vi "failUnlessXmlParsedCorrectly.vi"(4 "Convert EOL? (TRUE)":bool=TRUE, 6 "message (\"\")":string, 8 "error in":errorcluster, 9 "Expected Data":variant, 10 "XML String":string, 11 "reference in":refnum<class "EasyXML_XML_Subset_Evaluations.lvclass">) -> (0 "error out":errorcluster, 2 "Produced Data":variant, 3 "reference in":refnum<class "EasyXML_XML_Subset_Evaluations.lvclass">)   [LabVIEW 2013, in "EasyXML_XML_Subset_Evaluations.lvclass"]
doc: "Tests whether an XML string input matches flattened XML output generated from an in data structure"
uses:
  EasyXML_XML_Subset_Evaluations.lvclass
panel:
  # "Copyright © 2007 James Kring, Inc. All rights reserved.\n\nAuthor: Jim Kring [jim.kring@jameskring.com]\n\nThis library is provided \"AS IS\" ,WITHOUT WARRANTIES OR \nCONDITIONS OF ANY KIND, either express or implied.\n\nJames Kring, Inc. -- http://www.jameskring.com"
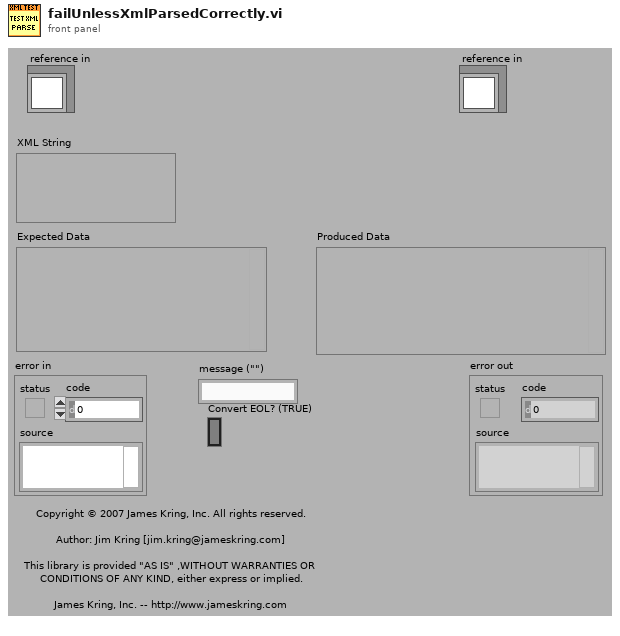
[diagram p1: front panel]
types:
  T1 = typedef "Type Descriptor__ogtk.ctl" = i16[]
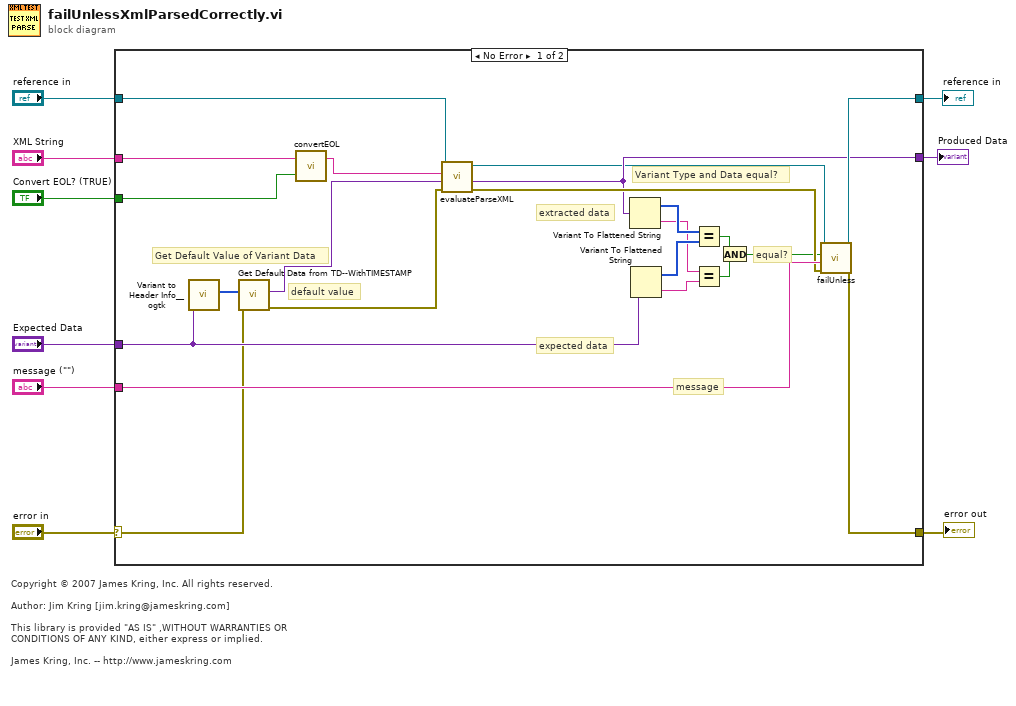
[diagram p0: block diagram]
diagram:
  # "Copyright © 2007 James Kring, Inc. All rights reserved.\n\nAuthor: Jim Kring [jim.kring@jameskring.com]\n\nThis library is provided \"AS IS\" ,WITHOUT WARRANTIES OR \nCONDITIONS OF ANY KIND, either express or implied.\n\nJames Kring, Inc. -- http://www.jameskring.com"
  n1 = case shown="No Error" "error in" {
    selector: "error in" -> [w12 w33]
    tunnel: [w26 w33] -> w8
    tunnel: [w28 w32] -> w6
    tunnel: "reference in" -> [w11 w32]
    tunnel: "message (\"\")" -> [w31 _]
    tunnel: "Expected Data" -> [w14 _]
    tunnel: "XML String" -> [w25 _]
    tunnel: [w22 _] -> w2
    tunnel: "Convert EOL? (TRUE)" -> [w23 _]
    frame No Error {
      # "Variant Type and Data equal?"
      # "message"
      # "equal?"
      # "expected data"
      # "extracted data"
      # "Get Default Value of Variant Data"
      # "default value"
      n2 = call <userlib>:"Variant to Header Info__ogtk.vi"("Variant"=w14) -> ("Type Descriptor"=w13:T1)  [unwired: 3 in, 2 out]
      n3 = call "Get Default Data from TD--WithTIMESTAMP.vi"("error in"=w12, "Type Descriptor"=w13) -> ("error out"=w30:errorcluster, "Default VData"=w29:variant)  [unwired: 8 in]
      n4 = call "convertEOL.vi"("Convert EOL? (TRUE)"=w23, "string"=w25) -> ("string out"=w24:string)  [unwired: 1 in]
      n5 = call-dynamic "evaluateParseXML.vi"("error in"=w30, "Default VData"=w29, "XML string"=w24, "reference in"=w11) -> ("error out"=w27:errorcluster, "LabVIEW Data"=w22:variant, "reference out"=w10:refnum<class "EasyXML_XML_Subset_Evaluations.lvclass">)  [unwired: 5 in]
      n6 = Variant To Flattened String(Variant=w22) -> (data string=w19:string, 1:w20:i16[])
      n7 = Variant To Flattened String(Variant=w14) -> (data string=w18:string, 1:w21:i16[])
      n8 = Equal?(x=w20, y=w21) -> (x = y?=w16:bool)
      n9 = Equal?(x=w19, y=w18) -> (x = y?=w17:bool)
      n10 = And(x=w16, y=w17) -> (x .and. y?=w15:bool)
      n11 = call-dynamic "failUnless.vi"("error in (no error)"=w27, "message (\"\")"=w31, "pass"=w15, "TestCase in"=w10) -> ("error out"=w26:errorcluster, "TestCase out"=w28:refnum<class "EasyXML_XML_Subset_Evaluations.lvclass">)  [unwired: 6 in]
    }
    frame Error {
    }
  }
  "error out" <- w8
  "reference in" <- w6
  "Produced Data" <- w2
